vi "DummyDataSimulation.vi"() -> ()   [LabVIEW 2020]
uses:
  StateGPSUpdate.ctl
  <vilib>/Skyline/Configuration/Configuration HTTP_class/NI Skyline Configuration HTTP.lvclass/NI Skyline Configuration HTTP.ctl
  TestData.ctl
  <vilib>/Skyline/Message/NI Skyline Message.lvclass
  <vilib>/Skyline/Configuration/Configuration HTTP_class/Open Configuration HTTP.vi
  <vilib>/Skyline/Message/HTTP Wrapper/NI Skyline Message HTTP.lvclass
  C:/Program Files (x86)/National Instruments/LabVIEW 2020/vi.lib/Skyline/Message/NI Skyline Message.lvclass
  <vilib>/Skyline/Configuration/HTTP/Open Configuration (Desktop).vi
  <vilib>/Skyline/Message/HTTP Wrapper/Open (HTTP).vi
  <vilib>/Skyline/Configuration/Configuration HTTP_class/NI Skyline Configuration HTTP.lvclass
  <vilib>/Skyline/Tag/Wrapper/Wrapper_class/NI Skyline Tag.lvclass
  <instrlib>/niSync/niSync.llb/niSync Read Last GPS or IRIG Timestamp (GPS).vi
  <vilib>/Skyline/Tag/Wrapper/Wrapper HTTP_class/Open Tag HTTP.vi
  <vilib>/Skyline/Tag/Wrapper/Wrapper HTTP_class/NI Skyline Tag HTTP.lvclass
  <vilib>/Skyline/Tag/Wrapper/Wrapper_class/Generate Tag Cluster (Boolean) 2.vi
  <vilib>/Skyline/Tag/Wrapper/Wrapper_class/Generate Tag Cluster (DBL) 2.vi
  <vilib>/Skyline/Tag/Wrapper/Wrapper_class/Generate Tag Cluster (Timestamp) 2.vi
  <vilib>/Skyline/Configuration/Configuration_class/NI Skyline Configuration.lvclass
  <vilib>/Skyline/Utilities/NI Skyline Utilities.lvlib
  <vilib>/Skyline/Tag/Wrapper/Wrapper_class/Delete Tag (Single).vi
panel:
  in  "SimulateOrHardware":bool
  in  "Resource Name":tag
  out "Percent Complete of Self Survey":i32
  out "Satellites Available":i32
  out "Mobile Mode":bool
  out "Latitude":dbl caption="latitude"
  out "Longitude":dbl caption="longitude"
  out "Altitude":dbl caption="altitude"
  in  "Stop":bool
  out "Current GPS Time":timestamp caption="time" format="%<%.9X\n%x>T"
  out "Warning Message":enum32{"Hide Warning", "Show Warning"}(tab)
  out "East Velocity":dbl
  out "North Velocity":dbl
  out "Up Velocity":dbl
  out "GPS time":timestamp
  out "timestamp":timestamp
  # "Warning: No external GPS antenna is present. \nYou may not be receiving valid location and velocity data."
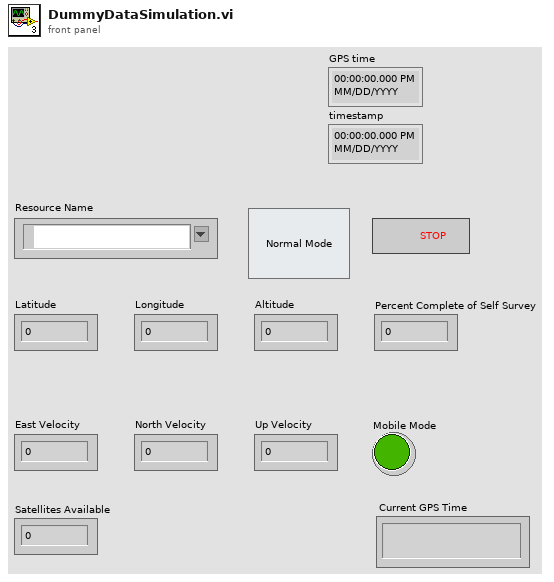
[diagram p1: front panel]
types:
  T1 = typedef "StateGPSUpdate.ctl" = enum16{"Init", "UpdateGPS", "Shutdown"}
  T2 = typedef "TestData.ctl" = cluster{"Latitude":dbl, "Longitude":dbl, "Timestamp":string, "TargetName":string, "MinionID":string}
  T3 = typedef "NI Skyline Tag.lvclass/Tag Value Cluster Wrapper.ctl" = cluster{"Configuration":refnum<class "NI Skyline Configuration.lvclass">, "Tag Cluster":T4}
  T4 = typedef "NI Skyline Tag.lvlib/Tag Value Cluster.ctl" = cluster{"Path":string, "Data Type":T5, "Value":string, "Time Stamp":timestamp}
  T5 = typedef "NI Skyline Tag.lvlib/DataType.ctl" = enum32{"Double", "I32", "String", "Boolean", "U64", "Timestamp"}
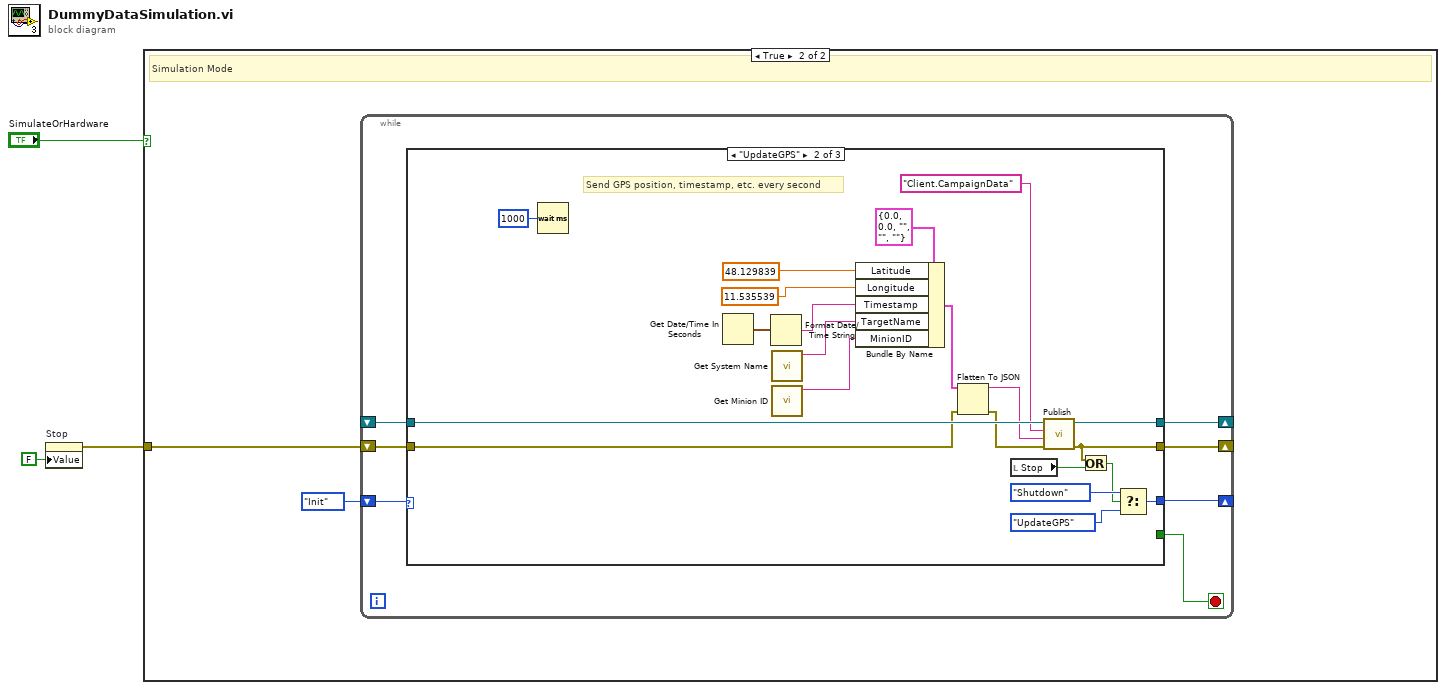
[diagram p0: block diagram]
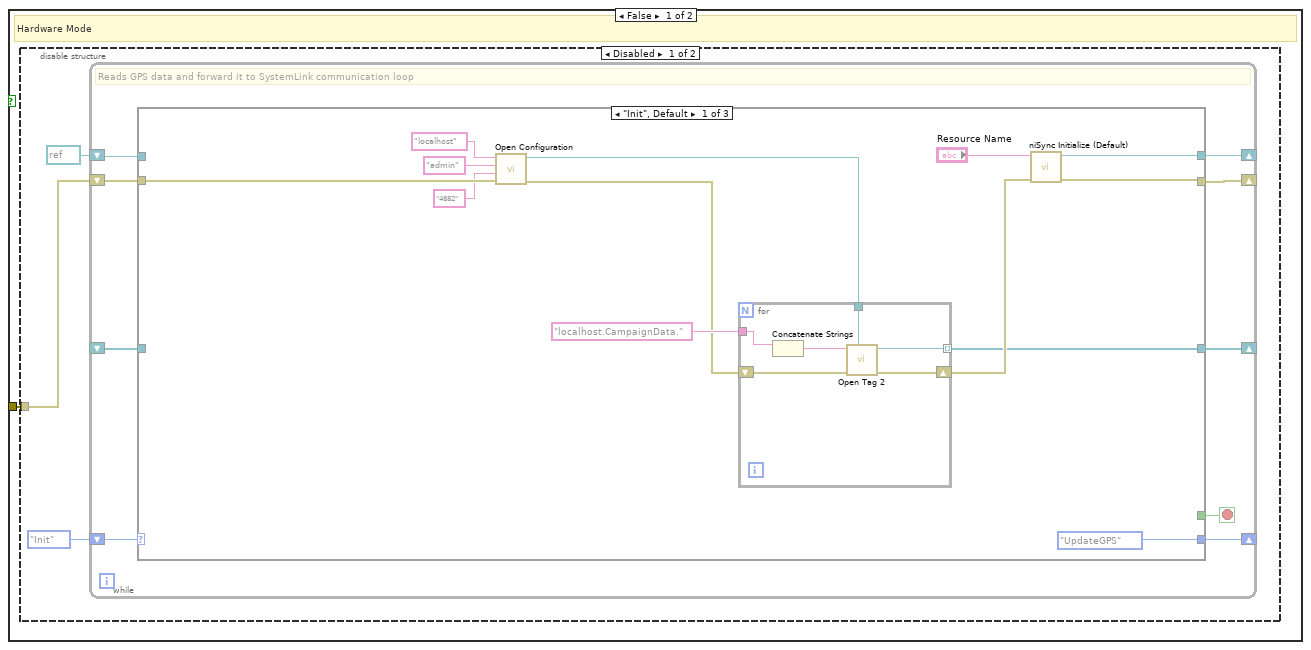
[diagram p2: hidden frame]
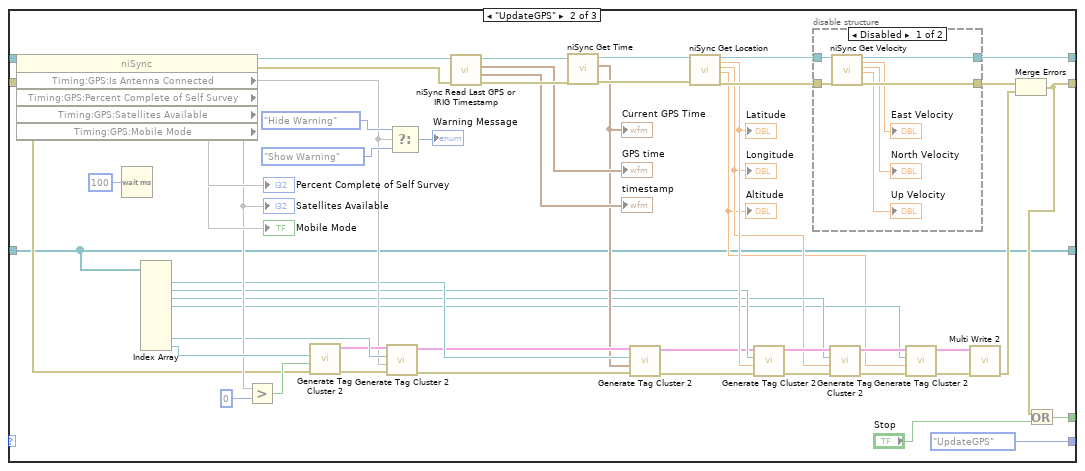
[diagram p3: hidden frame]
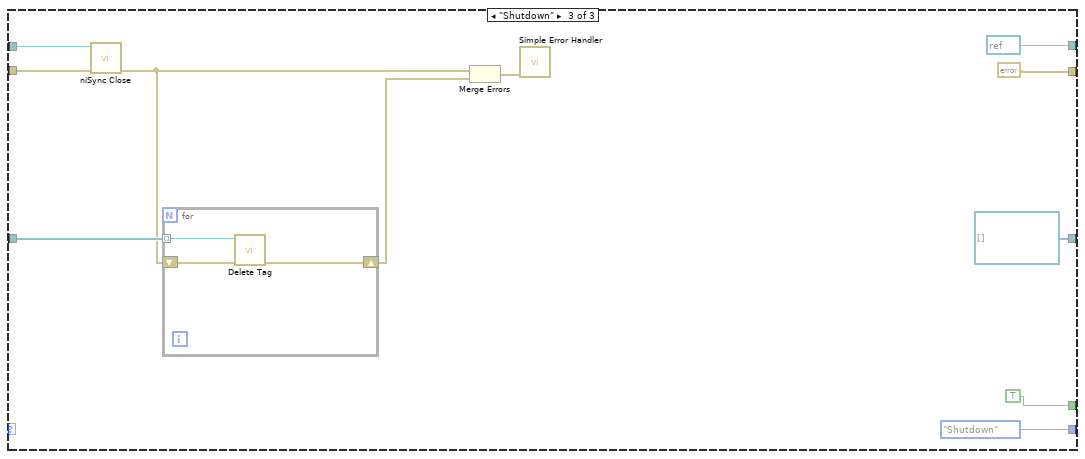
[diagram p5: hidden frame]
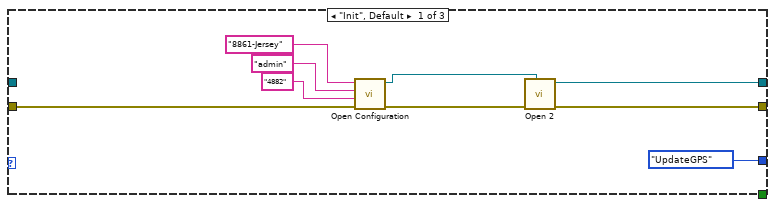
[diagram p7: hidden frame]
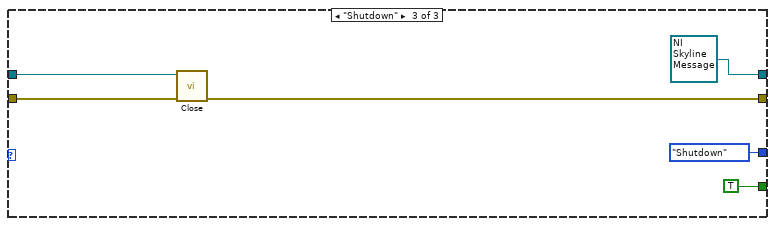
[diagram p8: hidden frame]
diagram:
  n1 = property on="Stop" class="Bool (strict)"("Value"=FALSE ("Stop")) -> (error out=w1:errorcluster)  [unwired: 2 in, 1 out]
  n2 = case shown="True" "SimulateOrHardware" {
    tunnel: w1 -> [w4 w111]
    frame False {
      # "Hardware Mode"
      n3 = disable-structure shown="Disabled" {
        disable-tunnel: w4 -> [w5 _]
        frame Disabled {
          n4 = while {
            shift-right: [w10] -> _
            shift-left: StateGPSUpdate."Init" -> [w11]
            shift-right: [w14] -> _
            shift-left: refnum<k15> refnum ("instrument handle out") -> [w16]
            shift-right: [w12] -> _
            shift-left: w5 -> [w15]
            shift-right: [w9] -> _
            shift-left: _ -> [w8]
            stop <- w13 stop-if-true
            # "Reads GPS data and forward it to SystemLink communication loop"
            n5 = case shown="\"Init\", Default" w11 {
              tunnel: w16 -> [_ w87 w107]
              tunnel: w15 -> [w22 w62 w106]
              tunnel: [w28 w84 refnum<k15> refnum ("instrument handle out")] -> w14
              tunnel: [_ w80 TRUE] -> w13
              tunnel: [w27 w37 errorcluster {"status"=FALSE, "code"=0, "source"=""} ("error out")] -> w12
              tunnel: [StateGPSUpdate."UpdateGPS" StateGPSUpdate."UpdateGPS" StateGPSUpdate."Shutdown"] -> w10
              tunnel: [w24 w36 refnum<class "NI Skyline Tag.lvclass">[] []] -> w9
              tunnel: w8 -> [_ w36 w101]
              frame "Init", Default {
                n6 = call-poly <vilib>:"Open Configuration.vi"("error in (no error)"=w22, "password"="4882", "username"="admin", "server url"="localhost") -> ("error out"=w21:errorcluster, "configuration"=w17:refnum<class "NI Skyline Configuration HTTP.lvclass">)  [unwired: 6 in]
                n7 = for {
                  tunnel: [w34] -> w24 mode=indexing
                  shift-right: [w35] -> w25
                  shift-left: w21 -> [w30]
                  tunnel: "localhost.CampaignData." -> [w32]
                  tunnel: w17 -> [w31]
                  n8 = Concatenate Strings(w32) -> (w33:string)  [unwired: 1 in]
                  n9 = call-poly <vilib>:"Open Tag 2.vi"("configuration"=w31, "error in (no error)"=w30, "path"=w33) -> ("error out"=w35:errorcluster, "tag"=w34:refnum<class "NI Skyline Tag.lvclass">)  [unwired: 7 in]
                }
                n10 = call <instrlib>:"niSync Initialize (Default).vi"("error in (no error)"=w25, "resource name"="Resource Name") -> ("error out"=w27:errorcluster, "instrument handle out"=w28:refnum<k15>)  [unwired: 8 in]
              }
              frame "UpdateGPS" {
                n11 = property class="niSync"(reference=w87, error in=w62) -> (reference out=w74:refnum<k15>, error out=w73:errorcluster, "Timing:GPS:Is Antenna Connected"=w58, "Timing:GPS:Percent Complete of Self Survey"=→"Percent Complete of Self Survey", "Timing:GPS:Satellites Available"=w64, "Timing:GPS:Mobile Mode"=→"Mobile Mode")
                "Satellites Available" <- w64
                n12 = Wait (ms)(milliseconds to wait=u32 100 ("millisecond multiple")) -> ()  [unwired: 1 out]
                n13 = Index Array(array=w36) -> (element #1=w57:refnum<class "NI Skyline Tag.lvclass">, element #2=w52:refnum<class "NI Skyline Tag.lvclass">, element #3=w47:refnum<class "NI Skyline Tag.lvclass">, element #4=w43:refnum<class "NI Skyline Tag.lvclass">, element #8=w61:refnum<class "NI Skyline Tag.lvclass">, element #9=w66:refnum<class "NI Skyline Tag.lvclass">)  [unwired: 9 in, 3 out]
                n14 = Greater?(x=w64, y=0) -> (0:w65:bool)
                n15 = call-poly <vilib>:"Generate Tag Cluster 2.vi"("error in (no error)"=w62, "value"=w65, "tag in"=w66) -> ("error out"=w59:errorcluster, "tag clusters out"=w60:T3[])  [unwired: 6 in, 1 out]
                n16 = call-poly <vilib>:"Generate Tag Cluster 2.vi"("error in (no error)"=w59, "value"=w58, "tag in"=w61, "tag clusters in"=w60) -> ("error out"=w55:errorcluster, "tag clusters out"=w56:T3[])  [unwired: 5 in, 1 out]
                n17 = Select(t=enum32{"Hide Warning", "Show Warning"}."Hide Warning" ("Warning Dialog"), s=w58, f=enum32{"Hide Warning", "Show Warning"}."Show Warning" ("Warning Dialog")) -> (s? t:f=→"Warning Message":enum32{"Hide Warning", "Show Warning"})
                n18 = call-poly <instrlib>:"niSync Read Last GPS or IRIG Timestamp.vi"("error in (no error)"=w73, "instrument handle"=w74) -> ("error out"=w71:errorcluster, "timestamp"=→"timestamp":timestamp, "GPS time"=→"GPS time":timestamp, "instrument handle out"=w72:refnum<k15>)  [unwired: 6 in]
                n19 = call <instrlib>:"niSync Get Time.vi"("error in (no error)"=w71, "instrument handle"=w72) -> ("error out"=w78:errorcluster, "time"=w54:timestamp, "instrument handle out"=w79:refnum<k15>)  [unwired: 5 in]
                "Current GPS Time" <- w54
                n20 = call-poly <vilib>:"Generate Tag Cluster 2.vi"("error in (no error)"=w55, "value"=w54, "tag in"=w57, "tag clusters in"=w56) -> ("error out"=w51:errorcluster, "tag clusters out"=w50:T3[])  [unwired: 5 in, 1 out]
                n21 = call <instrlib>:"niSync Get Location.vi"("instrument handle"=w79, "error in (no error)"=w78) -> ("instrument handle out"=w83:refnum<k15>, "latitude"=w53:dbl, "longitude"=w46:dbl, "altitude"=w42:dbl, "error out"=w82:errorcluster)  [unwired: 13 in]
                "Latitude" <- w53
                "Longitude" <- w46
                "Altitude" <- w42
                n22 = call-poly <vilib>:"Generate Tag Cluster 2.vi"("error in (no error)"=w51, "value"=w53, "tag in"=w52, "tag clusters in"=w50) -> ("error out"=w49:errorcluster, "tag clusters out"=w48:T3[])  [unwired: 5 in, 1 out]
                n23 = disable-structure shown="Disabled" {
                  disable-tunnel: [w94 w96] -> w84
                  disable-tunnel: [w93 w95] -> w38
                  disable-tunnel: w83 -> [w92 w96]
                  disable-tunnel: w82 -> [w91 w95]
                  frame Disabled {
                    n24 = call <instrlib>:"niSync Get Velocity.vi"("instrument handle"=w92, "error in (no error)"=w91) -> ("instrument handle out"=w94:refnum<k15>, "east velocity"=→"East Velocity":dbl, "north velocity"=→"North Velocity":dbl, "up velocity"=→"Up Velocity":dbl, "error out"=w93:errorcluster)  [unwired: 13 in]
                  }
                  frame Enabled {
                  }
                }
                n25 = call-poly <vilib>:"Generate Tag Cluster 2.vi"("error in (no error)"=w49, "value"=w46, "tag in"=w47, "tag clusters in"=w48) -> ("error out"=w45:errorcluster, "tag clusters out"=w44:T3[])  [unwired: 5 in, 1 out]
                n26 = call-poly <vilib>:"Generate Tag Cluster 2.vi"("error in (no error)"=w45, "value"=w42, "tag in"=w43, "tag clusters in"=w44) -> ("error out"=w40:errorcluster, "tag clusters out"=w41:T3[])  [unwired: 5 in, 1 out]
                n27 = call <vilib>:"Multi Write 2.vi"("error in (no error)"=w40, "tag clusters"=w41) -> ("error out"=w39:errorcluster)  [unwired: 9 in]
                n28 = Merge Errors(w38, w39) -> (w37:errorcluster)
                n29 = Or(x=w37, y="Stop") -> (x .or. y?=w80:bool)
              }
              frame "Shutdown" {
                n30 = call <instrlib>:"niSync Close.vi"("error in (no error)"=w106, "instrument handle"=w107) -> ("error out"=w97:errorcluster)  [unwired: 9 in]
                n31 = for {
                  tunnel: w101 -> [w110] mode=indexing
                  shift-right: [w109] -> w99
                  shift-left: w97 -> [w108]
                  n32 = call-poly <vilib>:"Delete Tag.vi"("error in (no error)"=w108, "tag"=w110) -> ("error out"=w109:errorcluster)  [unwired: 9 in]
                }
                n33 = Merge Errors(w97, w99) -> (w100:errorcluster)
                n34 = call <vilib>:"Simple Error Handler.vi"("error in (no error)"=w100) -> ()  [unwired: 4 in, 5 out]
              }
            }
          }
        }
        frame Enabled {
        }
      }
    }
    frame True {
      # "Simulation Mode"
      n35 = while {
        shift-right: [w118] -> _
        shift-left: w111 -> [w115]
        shift-right: [w116] -> _
        shift-left: StateGPSUpdate."Init" -> [w119]
        shift-right: [w117] -> _
        shift-left: _ -> [w113]
        stop <- w114 stop-if-true
        n36 = case shown="\"UpdateGPS\"" w119 {
          tunnel: [w123 w149 w151] -> w118
          tunnel: [w122 w142 refnum<class "NI Skyline Message.lvclass"> refnum ("message session out")] -> w117
          tunnel: [StateGPSUpdate."UpdateGPS" w147 StateGPSUpdate."Shutdown"] -> w116
          tunnel: w115 -> [w120 w133 w152]
          tunnel: [_ _ TRUE] -> w114
          tunnel: w113 -> [_ w141 w153]
          frame "Init", Default {
            n37 = call-poly <vilib>:"Open Configuration.vi"("error in (no error)"=w120, "password"="4882", "username"="admin", "server url"="8861-Jersey") -> ("error out"=w124:errorcluster, "configuration"=w125:refnum<class "NI Skyline Configuration HTTP.lvclass">)  [unwired: 6 in]
            n38 = call-poly <vilib>:"Open 2.vi"("configuration"=w125, "error in (no error)"=w124) -> ("error out"=w123:errorcluster, "message session"=w122:refnum<class "NI Skyline Message HTTP.lvclass">)  [unwired: 8 in]
          }
          frame "UpdateGPS" {
            # "Send GPS position, timestamp, etc. every second"
            n39 = Wait (ms)(milliseconds to wait=u32 1000) -> ()  [unwired: 1 out]
            n40 = Get Date/Time In Seconds() -> (seconds since 1Jan1904=w136:timestamp)
            n41 = Format Date/Time String(seconds (now)=w136) -> (date/time string=w135:string)  [unwired: 2 in]
            n42 = call <vilib>:"Get System Name.vi"() -> ("system name"=w130:string)  [unwired: 11 in]
            n43 = call <vilib>:"Get Minion ID.vi"() -> ("minion id"=w129:string)  [unwired: 11 in]
            n44 = Bundle By Name(cluster=T2 {"Latitude"=0.0, "Longitude"=0.0, "Timestamp"="", "TargetName"="", "MinionID"=""}, "Latitude"=48.129839, "Longitude"=11.535539, "Timestamp"=w135, "TargetName"=w130, "MinionID"=w129) -> (w134:T2)
            n45 = Flatten To JSON(anything=w134, error in (no error)=w133) -> (JSON string=w137:string, 11:w132:errorcluster)  [unwired: 1 in]
            n46 = local read "Stop"() -> (w143:bool)
            n47 = call-dynamic "Publish.vi"("error in (no error)"=w132, "message"=w137, "topic"="Client.CampaignData", "message session in"=w141) -> ("error out"=w149:errorcluster, "message session out"=w142:refnum<class "NI Skyline Message.lvclass">)  [unwired: 6 in]
            n48 = Or(x=w149, y=w143) -> (x .or. y?=w144:bool)
            n49 = Select(t=StateGPSUpdate."Shutdown", s=w144, f=StateGPSUpdate."UpdateGPS") -> (s? t:f=w147:T1)
          }
          frame "Shutdown" {
            n50 = call-dynamic "Close.vi"("error in (no error)"=w152, "message session"=w153) -> ("error out"=w151:errorcluster)  [unwired: 9 in]
          }
        }
      }
    }
  }
